vi "Look for (Label) Decoration.vi"(8 "error in":errorcluster, 9 "Decoration Content":string, 11 "VI  Ref":refnum<vi>) -> (0 "error out":errorcluster, 1 "Decoration Found?":bool, 3 "VI  Ref (dup)":refnum<vi>)   [LabVIEW 2021, in "Utilities.lvlib"]
doc: "Finds decorations in the diagram and looks for those containing the <B>Label</B> string as their first line.\n\nIf found, the decoration's content is replaced by <B>New Content</B>.\n\nNote that the comparison casts both label and content to lowercase characters."
uses:
  Utilities.lvlib
panel:
  # "see the AlliGator License on the block diagram (Ctrl+E or Window:Show Block Diagram)"
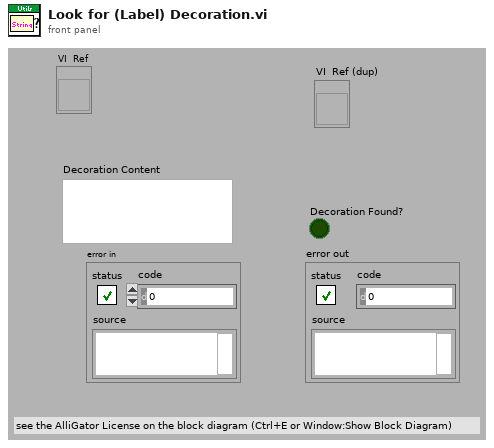
[diagram p1: front panel]
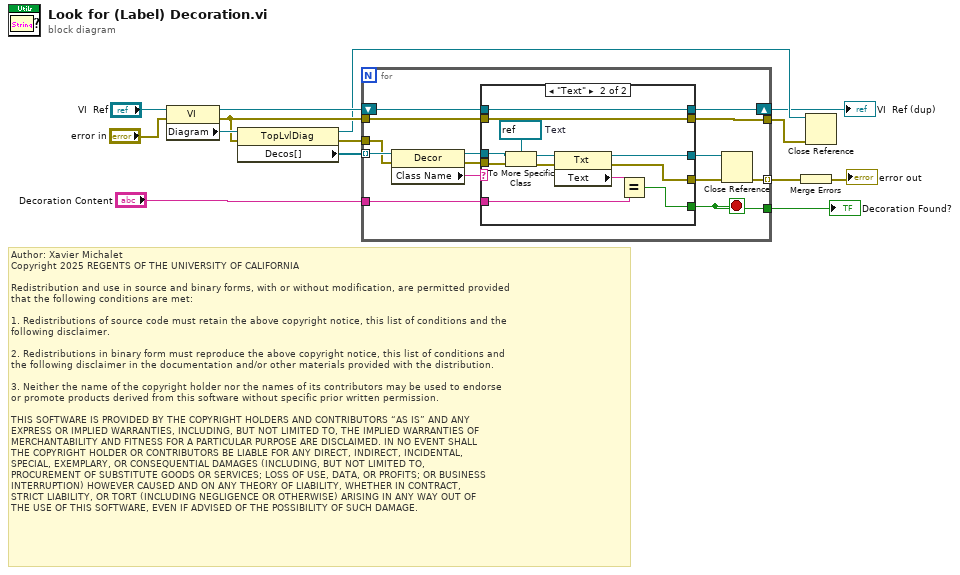
[diagram p0: block diagram]
diagram:
  # "Author: Xavier Michalet\nCopyright 2025 REGENTS OF THE UNIVERSITY OF CALIFORNIA\n\nRedistribution and use in source and binary forms, with or without modification, are permitted provided\nthat the following conditions are met:\n\n1. Redistributions of source code must retain the above copyright notice, this list of conditions and the\nfollowing disclaimer.\n\n2. Redistributions in binary form must reproduce the above copyright notice, this list of conditions and\nthe following disclaimer in the documentation and/or other materials provided with the distribution.\n\n3. Neither the name of the copyright holder nor the names of its contributors may be used to endorse \nor promote products derived from this software without specific prior written permission.\n\nTHIS SOFTWARE IS PROVIDED BY THE COPYRIGHT HOLDERS AND CONTRIBUTORS “AS IS” AND ANY \nEXPRESS OR IMPLIED WARRANTIES, INCLUDING, BUT NOT LIMITED TO, THE IMPLIED WARRANTIES OF\nMERCHANTABILITY AND FITNESS FOR A PARTICULAR PURPOSE ARE DISCLAIMED. IN NO EVENT SHALL\nTHE COPYRIGHT HOLDER OR CONTRIBUTORS BE LIABLE FOR ANY DIRECT, INDIRECT, INCIDENTAL, \nSPECIAL, EXEMPLARY, OR CONSEQUENTIAL DAMAGES (INCLUDING, BUT NOT LIMITED TO, \nPROCUREMENT OF SUBSTITUTE GOODS OR SERVICES; LOSS OF USE, DATA, OR PROFITS; OR BUSINESS\nINTERRUPTION) HOWEVER CAUSED AND ON ANY THEORY OF LIABILITY, WHETHER IN CONTRACT, \nSTRICT LIABILITY, OR TORT (INCLUDING NEGLIGENCE OR OTHERWISE) ARISING IN ANY WAY OUT OF\nTHE USE OF THIS SOFTWARE, EVEN IF ADVISED OF THE POSSIBILITY OF SUCH DAMAGE."
  n1 = property class="VI"(reference="VI  Ref", error in="error in") -> (reference out=w8:refnum<vi>, error out=w7:errorcluster, "Diagram"=w13:refnum<vi>)
  n2 = property class="TopLvlDiag"(reference=w13, error in=w7) -> (reference out=w5:refnum<vi>, error out=w12:errorcluster, "Decos[]"=w14:refnum<vi>[])
  n3 = for {
    tunnel: w14 -> [w23] mode=indexing
    tunnel: w12 -> [w18]
    tunnel: [w24] -> w11 mode=indexing
    tunnel: w7 -> [w20]
    tunnel: [w17] -> w3
    shift-right: [w19] -> w4
    shift-left: w8 -> [w21]
    tunnel: "Decoration Content" -> [w16]
    tunnel: [w15] -> w1
    stop <- w15 stop-if-true
    n4 = property class="Decor"(reference=w23, error in=w18) -> (reference out=w28:refnum<vi>, error out=w27:errorcluster, "Class Name"=w22:string)
    n5 = case shown="\"Text\"" w22 {
      tunnel: w28 -> [w32 w43]
      tunnel: w27 -> [w31 w44]
      tunnel: [w31 w36] -> w25
      tunnel: [w32 w35] -> w26
      tunnel: [_ w39] -> w15
      tunnel: w21 -> [w30 w34]
      tunnel: w20 -> [w29 w33]
      tunnel: [w30 w34] -> w19
      tunnel: [w29 w33] -> w17
      tunnel: w16 -> [_ w38]
      frame "", Default {
      }
      frame "Text" {
        w42 = refnum<vi> refnum  # Text
        n6 = To More Specific Class(target class=w42, reference=w43, error in=w44) -> (specific class reference=w41:refnum<vi>, error out=w40:errorcluster)
        n7 = property class="Txt"(reference=w41, error in=w40) -> (reference out=w35:refnum<vi>, error out=w36:errorcluster, "Text"=w37:string)
        n8 = Equal?(x=w37, y=w38) -> (x = y?=w39:bool)
      }
    }
    n9 = Close Reference(reference=w26, error in (no error)=w25) -> (error out=w24:errorcluster)
  }
  "Decoration Found?" <- w1
  "VI  Ref (dup)" <- w4
  n10 = Merge Errors(w11) -> (→"error out":errorcluster)
  n11 = Close Reference(reference=w5, error in (no error)=w3) -> ()  [unwired: 1 out]
